vi "1D limits response.vi"(7 "starting state":T2={"position (m)"=5.0, "velocity (m/s)"=10.0}, 11 "coefficient of restitution [0.9]":dbl=0.9 min=0.0 max=1.0 step=0.001, 13 "1D limits":T1={"lower (m)"=0.0, "upper (m)"=10.0}) -> (8 "ending state":T2={"position (m)"=5.0, "velocity (m/s)"=10.0})   [LabVIEW 2016]
doc: "This subVI handles the reflection off of the lower and upper limits of a box in 1D.\n\nPaul K Dixon\nP350\nCSUSB"
uses:
  typedef/1d state.ctl
  typedef/1d limits.ctl
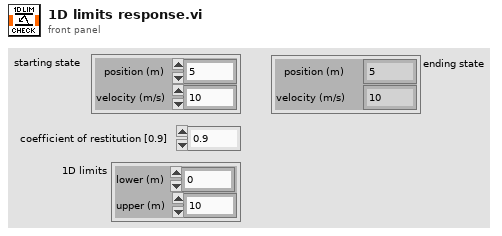
[diagram p1: front panel]
types:
  T1 = typedef "1d limits.ctl" = cluster{"lower (m)":dbl, "upper (m)":dbl}
  T2 = typedef "1d state.ctl" = cluster{"position (m)":dbl, "velocity (m/s)":dbl}
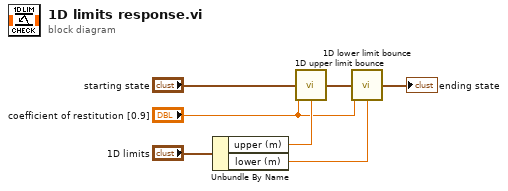
[diagram p0: block diagram]
diagram:
  n1 = Unbundle By Name("1D limits") -> ("upper (m)"=w4:dbl, "lower (m)"=w3:dbl)
  n2 = call "1D upper limit bounce.vi"("starting state"="starting state", "coefficient of restitution [0.9]"="coefficient of restitution [0.9]", "upper limit (m)"=w4) -> ("ending state"=w6:T2)  [unwired: 12 in]
  n3 = call "1D lower limit bounce.vi"("starting state"=w6, "coefficient of restitution [0.9]"="coefficient of restitution [0.9]", "lower limit (m)"=w3) -> ("ending state"=→"ending state":T2)  [unwired: 12 in]
